vi "4461DT-Acquire One.vi"(7 "AI Fs":dbl=192000.0 format="%#_13g") -> (4 "Stimulus":dbl[](array[numeric]), 8 "Array":dbl[](array[numeric]))   [LabVIEW 2015]
uses:
  Calibration VIs/Type Defs/Cal Stimulus.ctl
  <vilib>/DAQmx/write.llb/DAQmx Write (Analog 1D DBL 1Chan NSamp).vi
  <vilib>/DAQmx/read.llb/DAQmx Read (Analog 1D DBL 1Chan NSamp).vi
  <vilib>/DAQmx/create/channels.llb/DAQmx Create Channel (AO-Voltage-Basic).vi
  <vilib>/DAQmx/create/channels.llb/DAQmx Create Channel (AI-Voltage-Basic).vi
  <vilib>/DAQmx/configure/timing.llb/DAQmx Timing (Sample Clock).vi
  <vilib>/DAQmx/configure/trigger.llb/DAQmx Start Trigger (Digital Edge).vi
  <vilib>/DAQmx/miscellaneous.llb/DAQmx Fill In Error Info.vi
  <resource>/objmgr/daqmx.rc
panel:
  out "Graph":dbl[](graph)
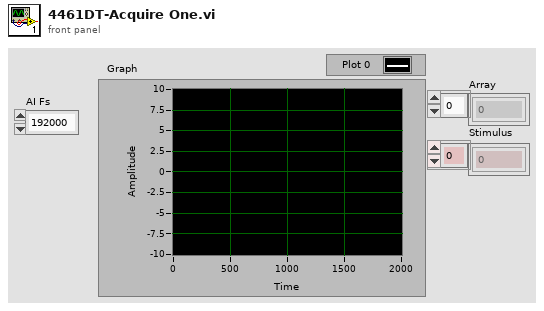
[diagram p1: front panel]
types:
  T1 = typedef "Cal Stimulus.ctl" = cluster{"Min Freq (Hz)":dbl, "Max Freq (Hz)":dbl, "Freq Step (Hz)":dbl, "Waveform":enum16{"Chirp", "Weighted"}, "Attenuation (dB)":dbl, "Sample Rate (Hz)":dbl}
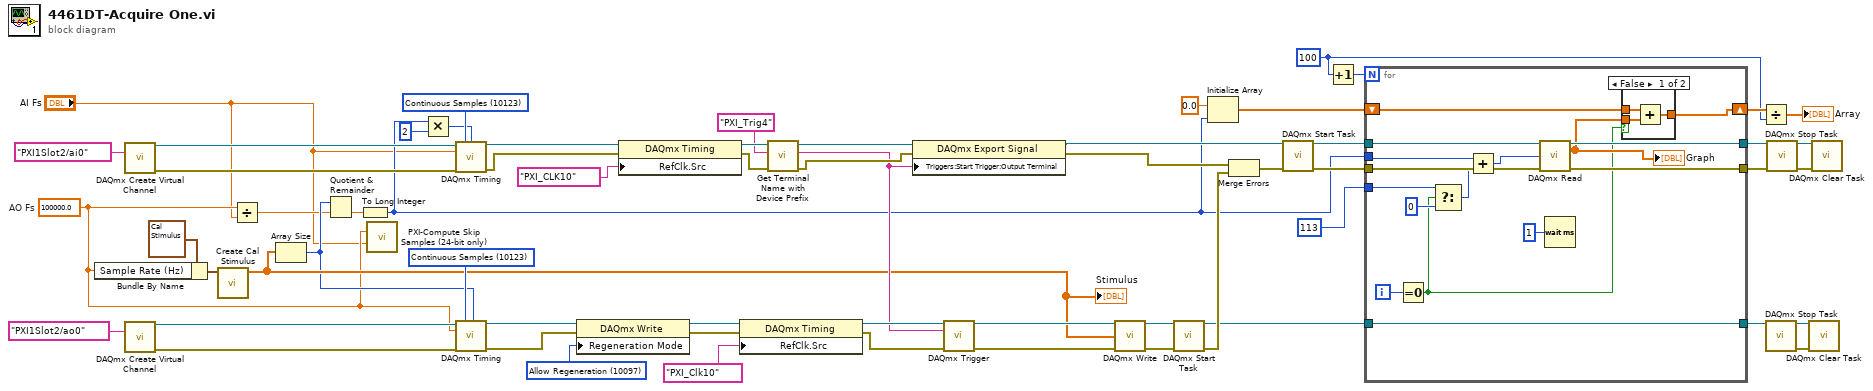
[diagram p0: block diagram]
diagram:
  w7 = 100
  w3 = 100000.0  # AO Fs
  w52 = 10123 items=["Finite Samples"=10178, "Continuous Samples"=10123, "Hardware Timed Single Point"=12522] ("sample mode")
  w55 = 10097 items=["Allow Regeneration"=10097, "Do Not Allow Regeneration"=10158] ("RegenMode")
  w59 = 10123 items=["Finite Samples"=10178, "Continuous Samples"=10123, "Hardware Timed Single Point"=12522] ("sample mode")
  n1 = Bundle By Name(cluster=T1 {"Min Freq (Hz)"=50.0, "Max Freq (Hz)"=50000.0, "Freq Step (Hz)"=50.0, "Waveform"=enum."Chirp", "Attenuation (dB)"=20.0, "Sample Rate (Hz)"=100000.0} ("Cal Stimulus"), "Sample Rate (Hz)"=w3) -> (w17:T1)
  n2 = call-poly <vilib>:"DAQmx Create Virtual Channel.vi"("physical channels"=tag "PXI1Slot2/ai0") -> ("task out"=w61:refnum<k21>, "error out"=w60:errorcluster)  [unwired: 13 in]
  n3 = call-poly <vilib>:"DAQmx Create Virtual Channel.vi"("physical channels"=tag "PXI1Slot2/ao0") -> ("task out"=w58:refnum<k21>, "error out"=w54:errorcluster)  [unwired: 13 in]
  n4 = call "Create Cal Stimulus.vi"("Cal Stimulus"=w17) -> ("Stimulus"=w16:dbl[])  [unwired: 8 in, 2 out]
  "Stimulus" <- w16
  n5 = Divide(x=w3, y="AI Fs") -> (x/y=w14:dbl)
  n6 = Array Size(array=w16) -> (size(s)=w15:i32)
  n7 = Quotient & Remainder(x=w15, y=w14) -> (floor(x/y)=w13:dbl)  [unwired: 1 out]
  n8 = To Long Integer(number=w13) -> (32bit integer=w12:i32)
  n9 = call "PXI-Compute Skip Samples (24-bit only).vi"("AO Sample Rate"=w3, "AI Sample Rate"="AI Fs") -> ()  [unwired: 13 in, 1 out]
  n10 = Multiply(x=w12, y=2) -> (x*y=w6:i32)
  n11 = call-poly <vilib>:"DAQmx Timing.vi"("task/channels in"=w61, "sample mode"=w59, "samples per channel"=w6, "rate"="AI Fs", "error in"=w60) -> ("task out"=w25:refnum<k21>, "error out"=w24:errorcluster)  [unwired: 9 in]
  n12 = call-poly <vilib>:"DAQmx Timing.vi"("task/channels in"=w58, "sample mode"=w52, "samples per channel"=w15, "rate"=w3, "error in"=w54) -> ("task out"=w56:refnum<k21>, "error out"=w57:errorcluster)  [unwired: 9 in]
  n13 = property class="DAQmx Write"(reference=w56, error in=w57, "Regeneration Mode"=w55) -> (reference out=w51:refnum<k21>, error out=w50:errorcluster)
  n14 = property class="DAQmx Timing"(reference=w25, error in=w24, "RefClk.Src"=tag "PXI_CLK10") -> (reference out=w21:refnum<k21>, error out=w22:errorcluster)
  n15 = property class="DAQmx Timing"(reference=w51, error in=w50, "RefClk.Src"=tag "PXI_Clk10") -> (reference out=w28:refnum<k21>, error out=w27:errorcluster)
  n16 = call "Get Terminal Name with Device Prefix.vi"("error in (no error)"=w22, "Local Terminal Name"="PXI_Trig4", "task/channels in"=w21) -> ("error out"=w30:errorcluster, "Terminal Name with Device Prefix"=w19:tag, "task out"=w29:refnum<k21>)  [unwired: 6 in]
  n17 = property class="DAQmx Export Signal"(reference=w29, error in=w30, "Triggers:Start Trigger:Output Terminal"=w19) -> (reference out=w33:refnum<k21>, error out=w32:errorcluster)
  n18 = call-poly <vilib>:"DAQmx Trigger.vi"("task/channels in"=w28, "source"=w19, "error in"=w27) -> ("task out"=w36:refnum<k21>, "error out"=w37:errorcluster)  [unwired: 11 in]
  n19 = call-poly <vilib>:"DAQmx Write.vi"("task/channels in"=w36, "data"=w16, "error in"=w37) -> ("task out"=w35:refnum<k21>, "error out"=w34:errorcluster)  [unwired: 10 in, 1 out]
  n20 = call <vilib>:"DAQmx Start Task.vi"("task/channels in"=w35, "error in"=w34) -> ("task out"=w45:refnum<k21>, "error out"=w49:errorcluster)  [unwired: 12 in]
  n21 = Initialize Array(0.0 ("element"), w12) -> (w10:dbl[])
  n22 = Merge Errors(w32, w49) -> (w48:errorcluster)
  n23 = call <vilib>:"DAQmx Start Task.vi"("task/channels in"=w33, "error in"=w48) -> ("task out"=w46:refnum<k21>, "error out"=w47:errorcluster)  [unwired: 12 in]
  n24 = Increment(x=w7) -> (x+1=w4:i32)
  n25 = for {
    N: w4 -> [_]
    tunnel: w47 -> [w74]
    tunnel: w46 -> [w75]
    tunnel: w45 -> [w76]
    tunnel: [w73] -> w44
    tunnel: [w69] -> w43
    tunnel: [w76] -> w42
    tunnel: w12 -> [w67]
    shift-right: [w70] -> w9
    shift-left: w10 -> [w72]
    tunnel: 113 ("Skip Samples") -> [w65]
    i -> [w68]
    n26 = Equal To 0?(x=w68) -> (x = 0?=w62:bool)
    n27 = Select(t=w65, s=w62, f=0) -> (s? t:f=w64:i32)
    n28 = Add(x=w67, y=w64) -> (x+y=w66:i32)
    n29 = call-poly <vilib>:"DAQmx Read.vi"("task/channels in"=w75, "number of samples per channel"=w66, "error in"=w74) -> ("task out"=w73:refnum<k21>, "data"=w71:dbl[], "error out"=w69:errorcluster)  [unwired: 10 in]
    "Graph" <- w71
    n30 = Wait (ms)(milliseconds to wait=u32 1) -> ()  [unwired: 1 out]
    n31 = case shown="False" w62 {
      tunnel: w72 -> [w80 w81]
      tunnel: w71 -> [w79 _]
      tunnel: [w78 w81] -> w70
      frame False {
        n32 = Add(x=w80, y=w79) -> (x+y=w78:dbl[])
      }
      frame True {
      }
    }
  }
  n33 = Divide(x=w9, y=w7) -> (x/y=→"Array":dbl[])
  n34 = call <vilib>:"DAQmx Stop Task.vi"("task/channels in"=w42) -> ("task out"=w39:refnum<k21>, "error out"=w38:errorcluster)  [unwired: 13 in]
  n35 = call <vilib>:"DAQmx Stop Task.vi"("task/channels in"=w44, "error in"=w43) -> ("task out"=w41:refnum<k21>, "error out"=w40:errorcluster)  [unwired: 12 in]
  n36 = call <vilib>:"DAQmx Clear Task.vi"("task in"=w39, "error in"=w38) -> ()  [unwired: 13 in, 1 out]
  n37 = call <vilib>:"DAQmx Clear Task.vi"("task in"=w41, "error in"=w40) -> ()  [unwired: 13 in, 1 out]
